vi "NF87XX.get driver type.vi"(0 "i ref in":refnum<vi>, 5 "error in (no error)":errorcluster) -> (14 "i ref out":refnum<vi>, 17 "Driver Types":T1[](array[typedef]), 19 "error out":errorcluster)   [LabVIEW 2014, in "NF87XX.lvlib"]
doc: "Returns the driver type: \"1\" for 3-channel open loop driver, \"2\" for 1-channel closed loop driver, and writes the information top own attributes.\n\nauthor: Stefan Götte\ndata: 09-JAN-2007\n\n\nLicense Agreement for this software:\n\nCopyright (C)\nGesellschaft für Schwerionenforschung, GSI\nPlanckstr. 1\n64291 Darmstadt\nGermany\n\nContact: D.Beck@gsi.de \n\nThis program is free software; you can redistribute it and/or modify it under the terms of the GNU General Public License as published by the Free Software Foundation; either version 2 of the license, or (at your option) any later version.\n\nThis program is distributed in the hope that it will be useful, but WITHOUT ANY WARRANTY; without even the implied warranty of MERCHANTABILITY or FITNESS FOR A PARTICULAR PURPOSE. See the GNU General License for more details (http://www.gnu.org).\n\nGesellschaft für Schwerionenforschung, GSI\nPlanckstr. 1, 64291 Darmstadt, Germany\nFor all questions and ideas contact: M.Richter@gsi.de, H.Brand@gsi.de or D.Beck@gsi.de.\nLast update: 17-JUN-2004"
uses:
  NF87XX.lvlib
  NF87XX.driver Type.ctl
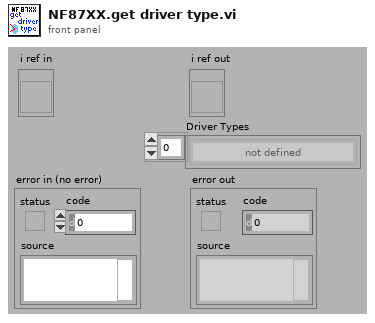
[diagram p1: front panel]
types:
  T1 = typedef "NF87XX.lvlib/NF87XX.driver Type.ctl" = enum16{"not defined", "3-ch open loop drv", "1-ch closed loop drv"}
  T2 = enum16{"User....", "DEF", "DIAG", "INI", "LOCK", "UNLOCK", "MAP", "SAV", "VER", "ACC", "CHL", "FOR", "GO", "HAL", "MOF", "MON", "MPV", "POS", "REL", "REV", "STA", "STO", "TYP", "VEL", "ABS", "SER", "NOS", "DRT", "FLI", "RLI", "FIN", "RIN", "AIN", "IN", "JOF", "JON", "OUT", "RES FINE", "RES COARSE", "02 (HEX)", "PWM", "CNT", "TMR", "HOSTNAME", "IPADDR", "IPMODE", "NETMASK", "GATEWAY", "DNSSRVR", "PASSWD", "ECHO", "MACADDR"}
  T3 = typedef "NF87XX.lvlib/NF87XX.i attribute.ctl" = cluster{"Con Settings":T4, "Drivers":T5[], "Status":cluster{"Service ID":i32, "Status":T7}, "Joystick available":bool, "VISA Resource":string}
  T4 = typedef "NewFocusPico - Driver np.lvlib/VISA & TCPIP Control.ctl" = cluster{"VISA or TCP/IP":bool, "Init Connection":bool, "Close Connection":bool, "Resource Name":refnum<visa-resource-name>, "hostname":string, "connection ID":refnum<k5>}
  T5 = typedef "NF87XX.lvlib/NF87XX.driver Settings.ctl" = cluster{"Name":string, "Driver Type":T1, "Pico Parameter type":T6, "Acceleration [Steps/s²]":cluster{"Motor 0":dbl, "Motor 1":dbl, "Motor 2":dbl}, "Start Velocity [Steps/s]":cluster{"Motor 0":dbl, "Motor 1":dbl, "Motor 2":dbl}, "Velocity [Steps/s]":cluster{"Motor 0":dbl, "Motor 1":dbl, "Motor 2":dbl}, "axis channel":i32, "Position":i32, "Position Service ID":i32}
  T6 = typedef "NewFocusPico - Driver np.lvlib/Pico Parameters.ctl" = cluster{"Pico Type":enum16{"Open-Loop Pico", "Close-Loop Pico", "Pico Ultra"}, "Acceleration (steps/sec^2)":string, "Velocity ( Hz)":string, "Driver":string, "Motor":string, "Channel":string, "Process Step":string}
  T7 = typedef "PH_StatusHandler.lvlib/PH_StatusHandler.Status.ctl" = i16
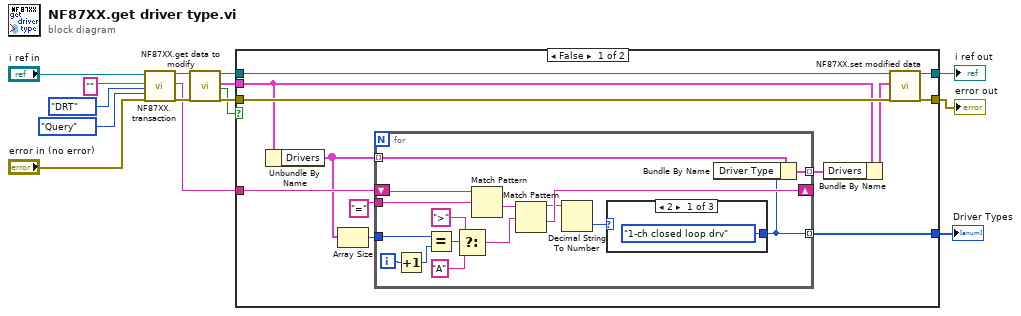
[diagram p0: block diagram]
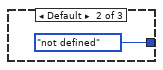
[diagram p2: hidden frame]
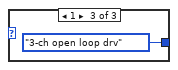
[diagram p3: hidden frame]
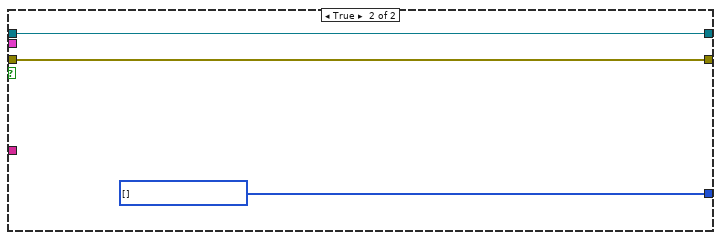
[diagram p4: hidden frame]
diagram:
  n1 = call "NF87XX.transaction.vi"("i ref in"="i ref in", "User Cmd/Numeric Argu"="", "MCL Cmd"=T2."DRT", "Query/Set"=enum16{"Query", "Set"}."Query", "error in (no error)"="error in (no error)") -> ("i ref out"=w10:refnum<vi>, "Read String"=w7:string, "error out"=w9:errorcluster)  [unwired: 12 in]
  n2 = call "NF87XX.get data to modify.vi"("i ref in"=w10, "error in (no error)"=w9) -> ("i ref out"=w3:refnum<vi>, "i attribute"=w8:T3, "timed out"=w1:bool, "error out"=w5:errorcluster)  [unwired: 14 in]
  n3 = case shown="False" w1 {
    tunnel: w8 -> [w18 _]
    tunnel: w7 -> [w26 _]
    tunnel: [w25 w47] -> w6
    tunnel: w5 -> [w24 w48]
    tunnel: [w23 w48] -> w4
    tunnel: w3 -> [w22 w49]
    tunnel: [w21 w49] -> w2
    frame False {
      n4 = Unbundle By Name(w18) -> ("Drivers"=w19:T5[])
      n5 = Array Size(array=w19) -> (size(s)=w20:i32)
      n6 = for {
        shift-right: [w34] -> _
        shift-left: w26 -> [w42]
        tunnel: [w29] -> w25 mode=indexing
        tunnel: "=" ("regular expression") -> [w41]
        tunnel: w20 -> [w31]
        tunnel: w19 -> [w30] mode=indexing
        tunnel: [w28] -> w17 mode=indexing
        i -> [w40]
        n7 = Increment(x=w40) -> (x+1=w39:i32)
        n8 = Equal?(x=w31, y=w39) -> (x = y?=w38:bool)
        n9 = Select(t=">", s=w38, f="A" ("regular expression")) -> (s? t:f=w37:string)
        n10 = Match Pattern(string=w42, regular expression=w41) -> (after substring=w43:string)  [unwired: 1 in, 3 out]
        n11 = Match Pattern(string=w43, regular expression=w37) -> (before substring=w32:string, after substring=w34:string)  [unwired: 1 in, 2 out]
        n12 = Decimal String To Number(string=w32) -> (number=w33:i32)  [unwired: 2 in, 1 out]
        n13 = case shown="2" w33 {
          tunnel: [NF87XX.driver_Type."1-ch closed loop drv" ("Driver Type") NF87XX.driver_Type."not defined" ("Driver Type") NF87XX.driver_Type."3-ch open loop drv" ("Driver Type")] -> w29
          frame 2 {
          }
          frame Default {
          }
          frame 1 {
          }
        }
        n14 = Bundle By Name(cluster=w30, "Driver Type"=w29) -> (w28:T5)
      }
      n15 = Bundle By Name(cluster=w18, "Drivers"=w17) -> (w16:T3)
      n16 = call "NF87XX.set modified data.vi"("i ref in"=w22, "i attribute"=w16, "error in (no error)"=w24) -> ("i ref out"=w21:refnum<vi>, "error out"=w23:errorcluster)  [unwired: 15 in]
    }
    frame True {
      w47 = T1[] [] items=["not defined", "3-ch open loop drv", "1-ch closed loop drv"]
    }
  }
  "error out" <- w4
  "i ref out" <- w2
  "Driver Types" <- w6
